vi "XY Graph Extrapolate Decay v2.vi"(0 "Plot in":cluster{"X Array":dbl[], "Y Array":dbl[]}, 1 "# Additional Points (-1: to Period)":i32, 5 "Head Fraction":dbl, 7 "Tail Fraction":dbl=0.5, 9 "Overweight Head (T)":bool=TRUE, 11 "Error In":errorcluster, 12 "Periodic Decay":bool, 13 "Shotnoise-limited? (T)":bool=TRUE, 14 "Period":dbl=0.5) -> (3 "Fitted Tau":dbl, 4 "Plot out":cluster{"X Array":dbl[], "Y Array":dbl[]}, 6 "# Additional Points":i32, 8 "Amplitude":dbl, 10 "Baseline":dbl, 15 "error out":errorcluster)   [LabVIEW 2021, in "XY Graph Add-Ons.lvlib"]
uses:
  XY Graph Add-Ons.lvlib
  Fits/Fit Statistics v2.ctl
  Fits/Convergence Criteria.ctl
  Fits/My Fit Stopping Criteria.ctl
  <vilib>/Analysis/6fits.llb/Curve Fitting Criteria.ctl
  Fits/Single Exponential/LM Single Exponential and gradient.vi
  <vilib>/gmath/statdist.llb/Gamma Random.vi
  Fits/Fits.lvlib
  <vilib>/Analysis/NI_AALPro.lvlib
  Math/Math.lvlib
  <vilib>/gmath/NI_Gmath.lvlib
panel:
  out "Plots":T1(graph)
  out "Fit Statistics":T2={"# Iterations"=0, "# Function Calls"=0, "Chi2"=0.0, "Chi2/DOF"=0.0, "Fit Convergence Criterion"=enum."Continue", "Gradient"=0.0, "|Delta Chi 2|"=0.0, "|Delta Chi 2|/Chi 2"=0.0, "Max |Delta a| /|a|"=0.0, "Lambda"=-1.0}
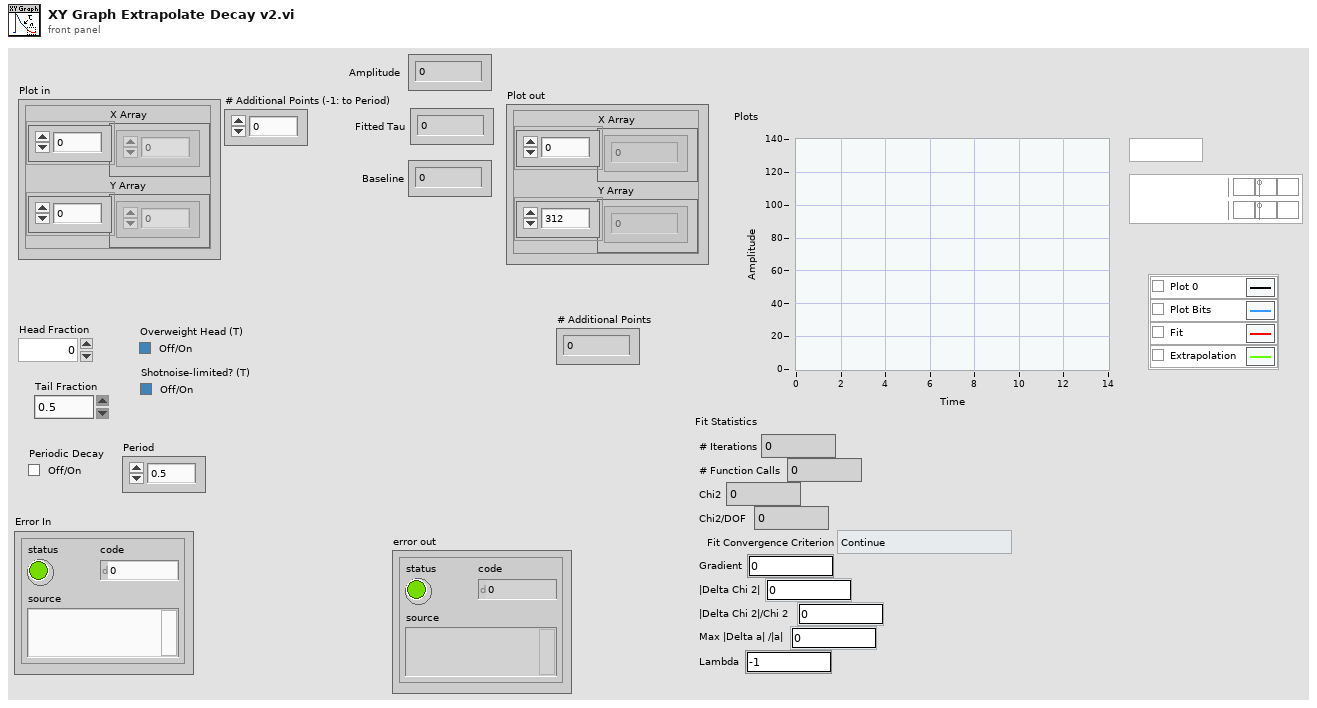
[diagram p1: front panel]
types:
  T1 = cluster{"X Array to Fit":dbl[], "best nonlinear fit":dbl[]}[]
  T2 = typedef "Fits.lvlib/Fit Statistics v2.ctl" = cluster{"# Iterations":i32, "# Function Calls":i32, "Chi2":dbl, "Chi2/DOF":dbl, "Fit Convergence Criterion":T3, "Gradient":dbl, "|Delta Chi 2|":dbl, "|Delta Chi 2|/Chi 2":dbl, "Max |Delta a| /|a|":dbl, "Lambda":dbl}
  T3 = typedef "Fits.lvlib/Convergence Criteria.ctl" = enum16{"Continue", "Tolerances Exceeded", "Max Time Exceeded", "Max Iterations Exceeded", "Max Function Evaluations Exceeded", "Scale Range Exceeded"}
  T4 = typedef "Fits.lvlib/My Fit Stopping Criteria.ctl" = cluster{"Max Iterations":i32, "Max Function Calls":i32, "Max Time":dbl[unit], "Function Tolerance":dbl, "Parameter Tolerance":dbl, "Gradient Tolerance":dbl, "Min Lambda":dbl, "Max Lambda":dbl, "Initial Tick Count":u32}
  T5 = cluster{"parameter minimum":dbl[], "parameter maximum":dbl[]}
  T6 = typedef "NI_AALPro.lvlib/Curve Fitting Criteria.ctl" = u16
  T7 = cluster{"Y Array to Fit":dbl[], "Y Array to Fit":dbl[]}
  T8 = cluster{"Y Array to Fit":dbl[], "best nonlinear fit":dbl[]}
  T9 = cluster{"Additional Tail Points":dbl[], "best nonlinear fit":dbl[]}[]
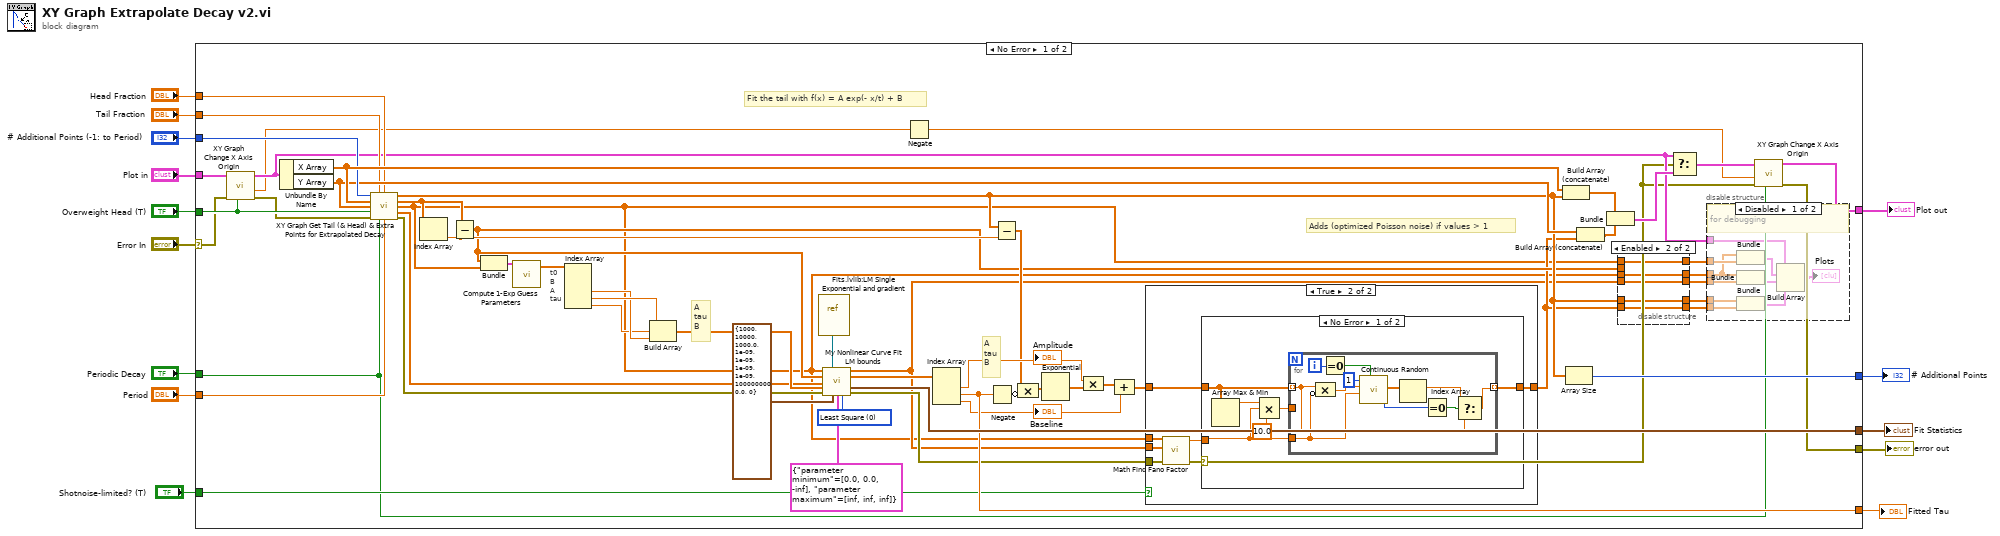
[diagram p0: block diagram]
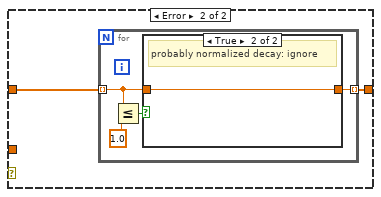
[diagram p3: hidden frame]
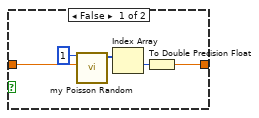
[diagram p4: hidden frame]
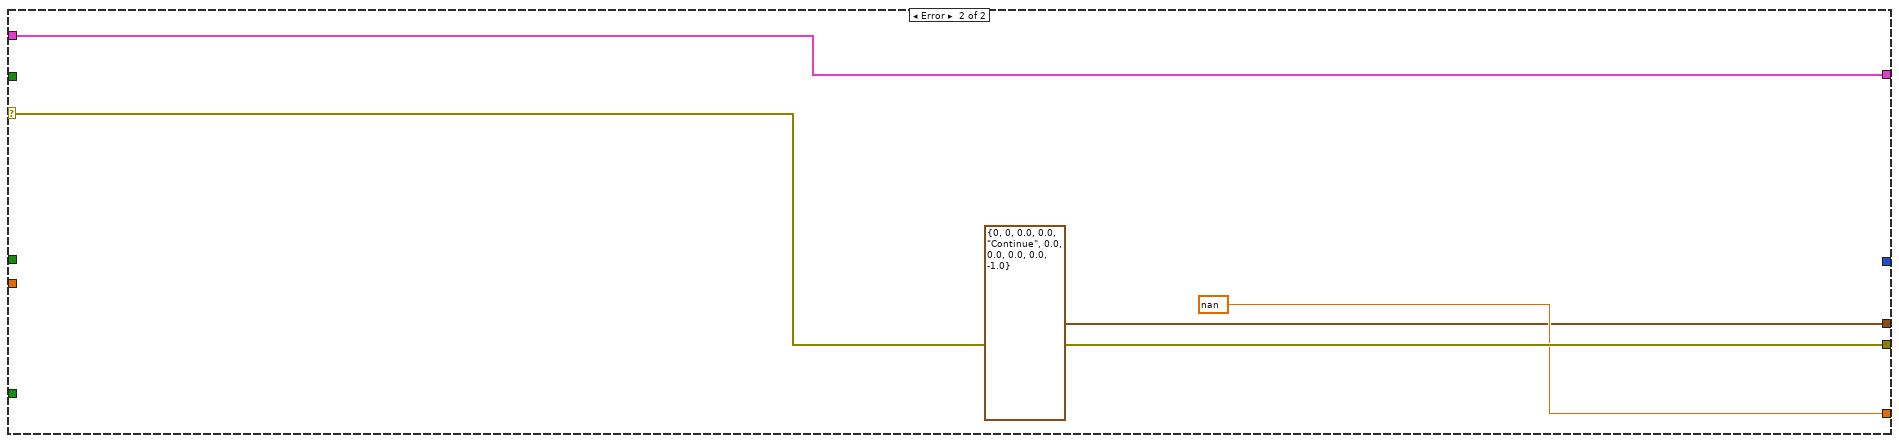
[diagram p7: hidden frame]
diagram:
  n1 = case shown="No Error" "Error In" {
    selector: "Error In" -> [w31 w131]
    tunnel: "# Additional Points (-1: to Period)" -> [w61 _]
    tunnel: "Tail Fraction" -> [w55 _]
    tunnel: [w72 T2 {"# Iterations"=0, "# Function Calls"=0, "Chi2"=0.0, "Chi2/DOF"=0.0, "Fit Convergence Criterion"=enum."Continue", "Gradient"=0.0, "|Delta Chi 2|"=0.0, "|Delta Chi 2|/Chi 2"=0.0, "Max |Delta a| /|a|"=0.0, "Lambda"=-1.0} ("Fit Statistics")] -> w12
    tunnel: [w27 w131] -> w11
    tunnel: [w69 nan ("Numeric")] -> w10
    tunnel: "Plot in" -> [w49 w130]
    tunnel: [w28 w130] -> w5
    tunnel: "Periodic Decay" -> [w26 _]
    tunnel: "Period" -> [w57 _]
    tunnel: "Head Fraction" -> [w51 _]
    tunnel: [w50 _] -> w3
    tunnel: "Overweight Head (T)" -> [w32 _]
    tunnel: "Shotnoise-limited? (T)" -> [w35 _]
    frame No Error {
      w20 = T6 0 items=["Least Square", "Least Absolute Residual", "Bisquare"] ("method")
      # "Adds (optimized Poisson noise) if values > 1"
      # "Fit the tail with f(x) = A exp(- x/t) + B"
      # "A\ntau\nB"
      # "t0\nB\nA\ntau"
      # "A\ntau\nB"
      n2 = call "XY Graph Change X Axis Origin.vi"("Shift (F)"=w32, "Error In"=w31, "Plot in"=w49) -> ("Error Out"=w30:errorcluster, "Shift"=w25:dbl, "Plot out"=w33:cluster{"X Array":dbl[], "Y Array":dbl[]})  [unwired: 6 in]
      n3 = Unbundle By Name(w33) -> ("X Array"=w62:dbl[], "Y Array"=w58:dbl[])
      n4 = call "XY Graph Get Tail (& Head) & Extra Points for Extrapolated Decay.vi"("# Additional Points"=w61, "Tail Fraction"=w55, "Head Fraction"=w51, "X Array"=w62, "Y Array"=w58, "Overweight Head"=w32, "Error In"=w30, "Periodic Decay"=w26, "Period"=w57) -> ("Additional Tail Points"=w44:dbl[], "X Array to Fit"=w18:dbl[], "Y Array to Fit"=w15:dbl[], "Weight Array"=w46:dbl[], "Error Out"=w56:errorcluster)  [unwired: 2 in]
      n5 = Index Array(array=w18) -> (element=w48:dbl)  [unwired: 1 in]
      n6 = Subtract(x=w18, y=w48) -> (x-y=w38:dbl[])
      n7 = Bundle(w38, "Y Array to Fit"=w15) -> (w19:cluster{dbl[], "Y Array to Fit":dbl[]})  [unwired: 1 in]
      n8 = call "Compute 1-Exp Guess Parameters.vi"("Decay"=w19) -> ("Guess Parameters"=w54:dbl[])  [unwired: 9 in, 1 out]
      n9 = Index Array(array=w54) -> (element #2=w45:dbl, element #3=w53:dbl, element #4=w34:dbl)  [unwired: 4 in, 1 out]
      n10 = Build Array(w53, w34, w45) -> (w52:dbl[])
      n11 = vi-ref "Fits.lvlib:LM Single Exponential and gradient.vi"() -> (w23:refnum<vi>)
      n12 = call "My Nonlinear Curve Fit LM bounds.vi"("Y"=w15, "f(x,a)"=w23, "X"=w38, "Weight"=w46, "initial parameters"=w52, "error in (no error)"=w56, "Termination Criteria"=T4 {"Max Iterations"=1000, "Max Function Calls"=10000, "Max Time"=1000.0, "Function Tolerance"=1e-09, "Parameter Tolerance"=1e-09, "Gradient Tolerance"=1e-09, "Min Lambda"=1e-09, "Max Lambda"=1000000000.0, "Initial Tick Count"=0}, "parameter bounds"=T5 {"parameter minimum"=[0.0, 0.0, -inf], "parameter maximum"=[inf, inf, inf]}, "NL Fit Method"=w20) -> ("best nonlinear fit"=w16:dbl[], "best fit parameters"=w67:dbl[], "Fit Statistics"=w72:T2, "error out"=w17:errorcluster)  [unwired: 1 in, 2 out]
      n13 = Negate(x=w25) -> (-x=w24:dbl)
      n14 = Index Array(array=w67) -> (element #1=w59:dbl, element #2=w69:dbl, element #3=w63:dbl)  [unwired: 3 in]
      "Amplitude" <- w59
      "Baseline" <- w63
      n15 = Negate(x=w69) -> (-x=w70:dbl)
      n16 = Subtract(x=w44, y=w48) -> (x-y=w47:dbl[])
      n17 = Compound Arithmetic op=MULTIPLY(w47, invert w70) -> (w68:dbl[])
      n18 = Exponential(1:w68) -> (0:w71:dbl[])
      n19 = Compound Arithmetic op=MULTIPLY(w59, w71) -> (w60:dbl[])
      n20 = Compound Arithmetic op=ADD(w60, w63) -> (w37:dbl[])
      n21 = case shown="True" w35 {
        tunnel: w37 -> [w73 w80]
        tunnel: [w73 w79] -> w36
        tunnel: w17 -> [_ w78]
        tunnel: w16 -> [_ w77]
        tunnel: w15 -> [_ w76]
        frame False {
        }
        frame True {
          n22 = call "Math Find Fano Factor.vi"("Error In"=w78, "Fitted Values"=w77, "Y Array"=w76) -> ("Error Out"=w75:errorcluster, "Fano Factor"=w74:dbl)  [unwired: 7 in]
          n23 = case shown="No Error" w75 {
            tunnel: w80 -> [w85 w99]
            tunnel: [w86 w98] -> w79
            tunnel: w74 -> [w83 _]
            frame No Error {
              n24 = Array Max & Min(array=w85) -> (max value=w84:dbl)  [unwired: 3 out]
              n25 = Compound Arithmetic op=MULTIPLY(w84, w83, 10.0 ("value")) -> (w81:dbl)
              n26 = for {
                tunnel: w83 -> [w87]
                tunnel: w85 -> [w89] mode=indexing
                tunnel: [w92] -> w86 mode=indexing
                tunnel: w81 -> [_]
                i -> [w91]
                n27 = Compound Arithmetic op=MULTIPLY(w89, invert w87) -> (w88:dbl)
                n28 = Equal To 0?(x=w91) -> (x = 0?=w90:bool)
                n29 = call-poly <vilib>:"Continuous Random.vi"("reset"=w90, "c"=w87, "b"=w88, "samples"=1) -> ("error"=w95:i32, "gamma random numbers"=w96:dbl[])  [unwired: 6 in]
                n30 = Index Array(array=w96) -> (element=w93:dbl)  [unwired: 1 in]
                n31 = Equal To 0?(x=w95) -> (x = 0?=w94:bool)
                n32 = Select(t=w93, s=w94, f=w89) -> (s? t:f=w92:dbl)
              }
            }
            frame Error {
              n33 = for {
                tunnel: w99 -> [w102] mode=indexing
                tunnel: [w103] -> w98 mode=indexing
                n34 = Less Or Equal?(x=w102, y=1.0) -> (x <= y?=w100:bool)
                n35 = case shown="True" w100 {
                  tunnel: [w105 w109] -> w103
                  tunnel: w102 -> [w104 w109]
                  frame False {
                    n36 = call "my Poisson Random.vi"("lambda"=w104, "samples (1)"=1 ("samples")) -> ("Poisson random data"=w107:i32[])  [unwired: 8 in, 1 out]
                    n37 = Index Array(array=w107) -> (element=w106:i32)  [unwired: 1 in]
                    n38 = To Double Precision Float(number=w106) -> (double precision float=w105:dbl)
                  }
                  frame True {
                    # "probably normalized decay: ignore"
                  }
                }
              }
            }
          }
        }
      }
      n39 = Build Array (concatenate)(w62, w44) -> (w66:dbl[])
      n40 = Array Size(array=w44) -> (size(s)=w50:i32)
      n41 = Build Array (concatenate)(w58, w36) -> (w65:dbl[])
      n42 = Bundle(w66, w65) -> (w64:cluster{dbl[], dbl[]})  [unwired: 1 in]
      n43 = disable-structure shown="Enabled" {
        disable-tunnel: w15 -> [w112 w115]
        disable-tunnel: w15 -> [_ w114]
        disable-tunnel: w16 -> [w111 w113]
        disable-tunnel: w44 -> [_ w117]
        disable-tunnel: w36 -> [_ w116]
        disable-tunnel: [_ w117] -> w43
        disable-tunnel: [_ w116] -> w42
        disable-tunnel: [w112 w115] -> w41
        disable-tunnel: [w110 w114] -> w40
        disable-tunnel: [w111 w113] -> w39
        disable-tunnel: w38 -> [w110 _]
        frame Disabled {
        }
        frame Enabled {
        }
      }
      n44 = Select(t=w33, s=w17, f=w64) -> (s? t:f=w29:cluster{"X Array":dbl[], "Y Array":dbl[]})
      n45 = disable-structure shown="Disabled" {
        disable-tunnel: w39 -> [w127 _]
        disable-tunnel: w40 -> [w119 _]
        disable-tunnel: w41 -> [w125 _]
        disable-tunnel: w42 -> [w122 _]
        disable-tunnel: w43 -> [w121 _]
        disable-tunnel: w33 -> [w118 _]
        frame Disabled {
          # "for debugging"
          n46 = Bundle("Y Array to Fit"=w119, "Y Array to Fit"=w125) -> (w124:T7)  [unwired: 1 in]
          n47 = Bundle("Y Array to Fit"=w119, "best nonlinear fit"=w127) -> (w126:T8)  [unwired: 1 in]
          n48 = Bundle("Additional Tail Points"=w121, w122) -> (w120:cluster{"Additional Tail Points":dbl[], dbl[]})  [unwired: 1 in]
          n49 = Build Array(w118, w124, w126, w120) -> (→"Plots":T9)
        }
        frame Enabled {
        }
      }
      n50 = call "XY Graph Change X Axis Origin.vi"("Shift (F)"=w26, "Error In"=w17, "New X Origin (0)"=w24, "Plot in"=w29) -> ("Error Out"=w27:errorcluster, "Plot out"=w28:cluster{"X Array":dbl[], "Y Array":dbl[]})  [unwired: 5 in, 1 out]
    }
    frame Error {
    }
  }
  "Fit Statistics" <- w12
  "error out" <- w11
  "Fitted Tau" <- w10
  "Plot out" <- w5
  "# Additional Points" <- w3
